vi "1 Channel 1 Sample - Auto Indexing.vi"() -> ()   [LabVIEW 2026, in "synnax_clib.lvlib"]
uses:
  lvlib/synnax_clib.lvlib
  lvlib/typedefs/connection_config.ctl
  lvlib/classes/Client/Private/synnax channel retrieve keys Single.vi
  lvlib/classes/Writer/Private/synnax writer open Single.vi
  lvlib/classes/Writer/Private/Writes/DBL/Write 1Ch 1Samp (DBL).vi
  lvlib/classes/Synnax Writer.lvclass
  lvlib/classes/Client/Synnax Client.lvclass
panel:
  out "cos(x)":dbl
  in  "Stop":bool
  in  "Channel":string="my_f64_chan"
  in  "Connection Config":T1={"host"="localhost", "port"=9090, "username"="synnax", "password"="seldon"}
  out "error out":errorcluster
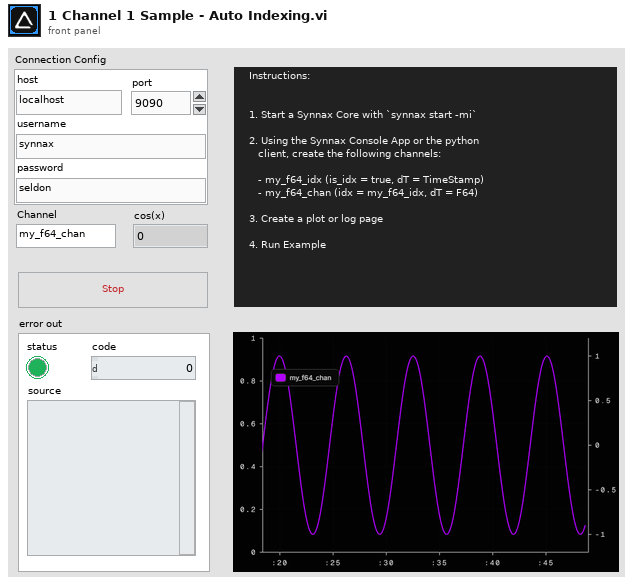
[diagram p1: front panel]
types:
  T1 = typedef "synnax_clib.lvlib/connection_config.ctl" = cluster{"host":string, "port":u16, "username":string, "password":string}
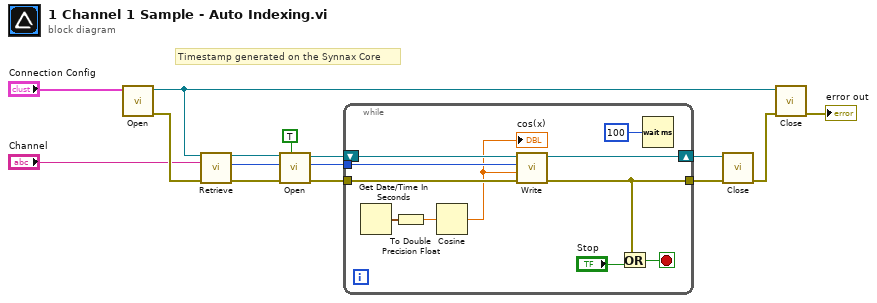
[diagram p0: block diagram]
diagram:
  # "Timestamp generated on the Synnax Core"
  n1 = call "Open.vi"("Connection Config"="Connection Config") -> ("error out"=w10:errorcluster, "Synnax Client out"=w12:refnum<class "Synnax Client.lvclass">)  [unwired: 9 in]
  n2 = call-poly "Retrieve.vi"("Synnax Client in"=w12, "channel name"="Channel", "error in"=w10) -> ("Synnax Client out"=w6:refnum<class "Synnax Client.lvclass">, "channel key"=w3:u32, "error out"=w14:errorcluster)  [unwired: 8 in, 2 out]
  n3 = call-poly "Open.vi"("auto_index (F)"=TRUE, "error in"=w14, "channel in"=w3, "Synnax Client in"=w6) -> ("error out"=w7:errorcluster, "channel out"=w4:u32, "writer out"=w9:refnum<class "Synnax Writer.lvclass">)  [unwired: 5 in]
  n4 = while {
    tunnel: w4 -> [w23]
    shift-right: [w25] -> w8
    shift-left: w9 -> [w26]
    tunnel: w7 -> [w24]
    tunnel: [w16] -> w15
    stop <- w17 stop-if-true
    n5 = Get Date/Time In Seconds() -> (seconds since 1Jan1904=w19:timestamp)
    n6 = To Double Precision Float(number=w19) -> (double precision float=w18:dbl)
    n7 = Cosine(x=w18) -> (cos(x)=w21:dbl)
    "cos(x)" <- w21
    n8 = call-poly "Write.vi"("error in"=w24, "data"=w21, "channel"=w23, "Writer"=w26) -> ("error out"=w16:errorcluster, "Writer Out"=w25:refnum<class "Synnax Writer.lvclass">)  [unwired: 6 in]
    n9 = Or(x=w16, y="Stop") -> (x .or. y?=w17:bool)
    n10 = Wait (ms)(milliseconds to wait=u32 100) -> ()  [unwired: 1 out]
  }
  n11 = call "Close.vi"("error in"=w15, "writer"=w8) -> ("error out"=w11:errorcluster)  [unwired: 9 in]
  n12 = call "Close.vi"("error in"=w11, "Synnax Client in"=w12) -> ("error out"=→"error out":errorcluster)  [unwired: 9 in]
